vi "SlowLogger_Setup.vi"(0 "SlowLogger in":refnum<class "SlowLogger.lvclass">, 1 "Category":string, 2 "Variable Name":string, 3 "Max Log Speed [Delta Time] (seconds)":dbl=10.0, 4 "Period to update history plots (seconds)\nUnset (65535) = Use MIDAS default in ODB\n0 = Record but do not put in histories":u16=65535, 5 "error in (no error)":errorcluster, 6 "Skip ODB on the way to \nhistories (fast, but no ALARMS possible)":bool, 7 "Equipment Description (32 chars)":string) -> (14 "SlowLogger out":refnum<class "SlowLogger.lvclass">, 19 "error out":errorcluster)   [LabVIEW 2018, in "feGEM DataPacker.lvlib" / "SlowLogger.lvclass"]
uses:
  SlowLogger.lvclass
  DataPacker/DataStructures/GEM_BANK_CLUSTER_typedef.ctl
  DataPacker/DataStructures/GEM_DATA_cluster_typedef.ctl
  SlowLogger.lvclass/SlowLogger.ctl
  feGEM DataPacker.lvlib
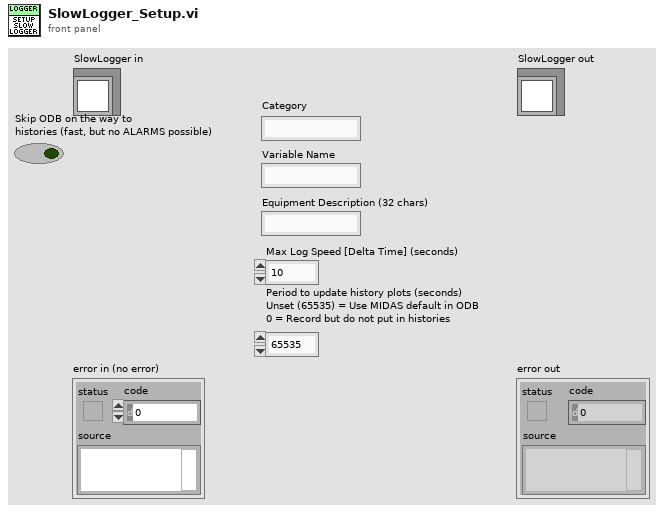
[diagram p1: front panel]
types:
  T1 = typedef "feGEM DataPacker.lvlib/GEM_BANK_CLUSTER_typedef.ctl" = cluster{"Category":string, "Variable Name":string, "Equipment description":string, "History Settings":u16, "Period to update history plots":u16, "GEM_DATA Cluster":T2}
  T2 = typedef "feGEM DataPacker.lvlib/GEM_DATA_cluster_typedef.ctl" = cluster{"DataType":string, "Formatted Data":u8[], "data byte order (Little Endian prefered)":enum16{"big-endian, network order", "native, host order", "little-endian"}}
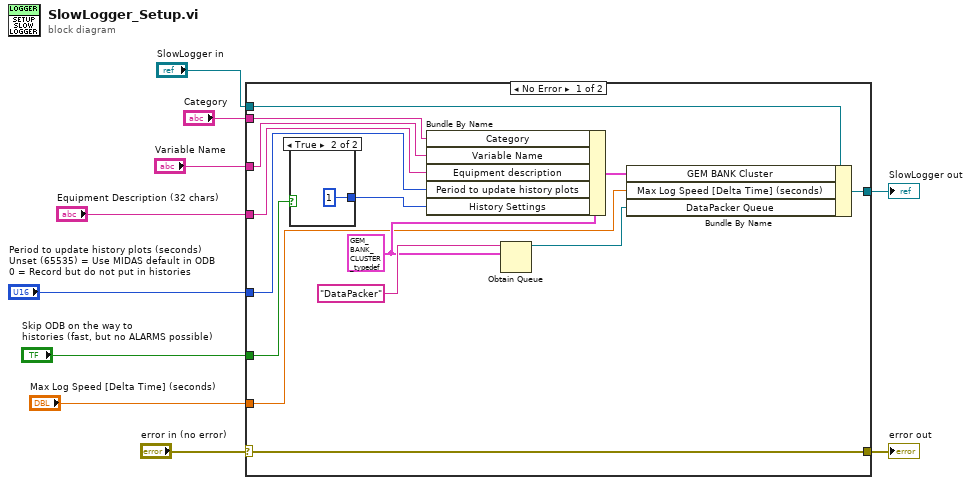
[diagram p0: block diagram]
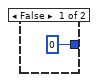
[diagram p2: hidden frame]
diagram:
  n1 = case shown="No Error" "error in (no error)" {
    selector: "error in (no error)" -> [w24 w27]
    tunnel: [w24 w27] -> w9
    tunnel: [w22 w28] -> w7
    tunnel: "SlowLogger in" -> [w23 w28]
    tunnel: "Category" -> [w19 _]
    tunnel: "Variable Name" -> [w18 _]
    tunnel: "Max Log Speed [Delta Time] (seconds)" -> [w14 _]
    tunnel: "Period to update history plots (seconds)\nUnset (65535) = Use MIDAS default in ODB\n0 = Record but do not put in histories" -> [w16 _]
    tunnel: "Equipment Description (32 chars)" -> [w17 _]
    tunnel: "Skip ODB on the way to \nhistories (fast, but no ALARMS possible)" -> [w12 _]
    frame No Error {
      w20 = T1 {"Category"="", "Variable Name"="", "Equipment description"="", "History Settings"=0, "Period to update history plots"=0, "GEM_DATA Cluster"={"DataType"="", "Formatted Data"=[], "data byte order (Little Endian prefered)"=enum."big-endian, network order"}} ("output cluster")
      n2 = case shown="True" w12 {
        tunnel: [u16 0 ("History Settings") u16 1 ("History Settings")] -> w11
        frame False {
        }
        frame True {
        }
      }
      n3 = Bundle By Name(cluster=w20, "Category"=w19, "Variable Name"=w18, "Equipment description"=w17, "Period to update history plots"=w16, "History Settings"=w11) -> (w15:T1)
      n4 = Obtain Queue(name (unnamed)="DataPacker", element data type=w20) -> (queue out=w13:refnum<queue>)  [unwired: 3 in, 2 out]
      n5 = Bundle By Name(cluster=w23, "GEM BANK Cluster"=w15, "Max Log Speed [Delta Time] (seconds)"=w14, "DataPacker Queue"=w13) -> (w22:refnum<class "SlowLogger.lvclass">)
    }
    frame Error {
    }
  }
  "error out" <- w9
  "SlowLogger out" <- w7
